vi "ELRecv.vi"(0 "connection ID":refnum<k16>) -> (2 "IP address":string, 3 "ELdata":T1, 4 "Error Out":errorcluster caption="エラー出力")   [LabVIEW 2017]
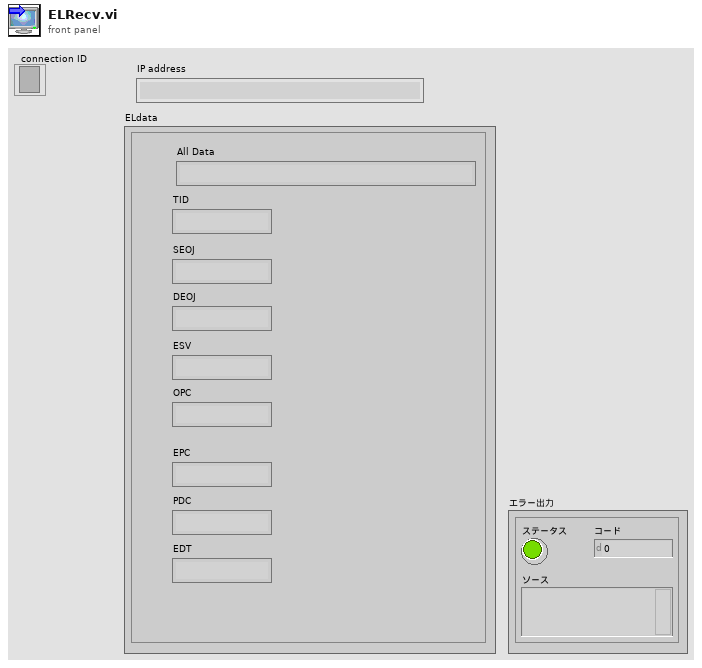
[diagram p1: front panel]
types:
  T1 = cluster{"All Data":string, "EPC":string, "EDT":string, "SEOJ":string, "DEOJ":string, "ESV":string, "OPC":string, "PDC":string, "TID":string}
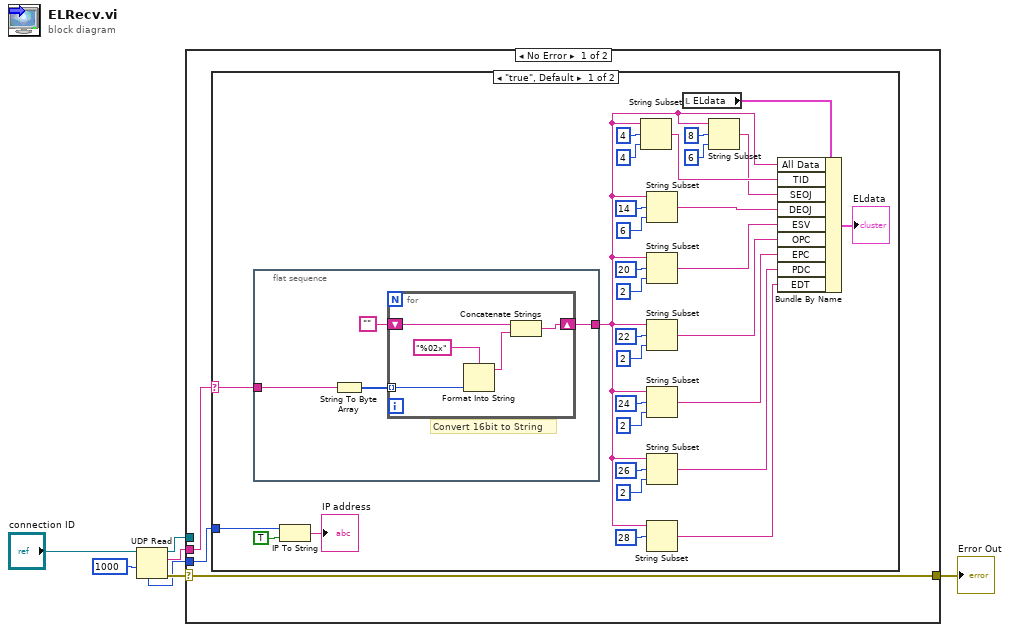
[diagram p0: block diagram]
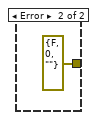
[diagram p3: hidden frame]
diagram:
  n1 = UDP Read(connection ID="connection ID", timeout ms (25000)=1000) -> (data out=w5:string, error out=w4:errorcluster, 3:w1:refnum<k16>, 6:w2:u32)  [unwired: 2 in, 1 out]
  n2 = case shown="No Error" w4 {
    selector: w4 -> [w8 _]
    tunnel: [w8 errorcluster {"status"=FALSE, "code"=0, "source"=""} ("error IO")] -> w3
    tunnel: w5 -> [w10 _]
    tunnel: w2 -> [w9 _]
    tunnel: w1 -> [_ _]
    frame No Error {
      n3 = case "ケースストラクチャ" shown="\"true\", Default" w10 {
        selector: w10 -> [w12 _]
        tunnel: w9 -> [w13 _]
        frame "true", Default {
          n4 = flat-sequence {
            tunnel: w12 -> [w42]
            tunnel: [w41] -> w11
            frame #0 {
              # "Convert 16bit to String"
              n5 = String To Byte Array(string=w42) -> (unsigned byte array=w43:u8[])
              n6 = for {
                tunnel: w43 -> [w48] mode=indexing
                shift-right: [w47] -> w41
                shift-left: "" -> [w45]
                n7 = Format Into String(format string="%02x" ("形式文字列"), w48) -> (resulting string=w46:string)  [unwired: 2 in, 1 out]
                n8 = Concatenate Strings(w45, w46) -> (w47:string)
              }
            }
          }
          n9 = IP To String(1:TRUE ("ドット表記法?（F）"), 2:w13) -> (0:→"IP address":string)
          n10 = String Subset(string=w11, offset (0)=4, length (rest)=4) -> (substring=w37:string)
          n11 = String Subset(string=w11, offset (0)=14, length (rest)=6) -> (substring=w33:string)
          n12 = String Subset(string=w11, offset (0)=20, length (rest)=2) -> (substring=w36:string)
          n13 = String Subset(string=w11, offset (0)=22, length (rest)=2) -> (substring=w34:string)
          n14 = String Subset(string=w11, offset (0)=24, length (rest)=2) -> (substring=w31:string)
          n15 = String Subset(string=w11, offset (0)=26, length (rest)=2) -> (substring=w35:string)
          n16 = String Subset(string=w11, offset (0)=28) -> (substring=w30:string)  [unwired: 1 in]
          n17 = local read "ELdata"() -> (w40:T1)
          n18 = String Subset(string=w11, offset (0)=8, length (rest)=6) -> (substring=w32:string)
          n19 = Bundle By Name(cluster=w40, "All Data"=w11, "TID"=w37, "SEOJ"=w32, "DEOJ"=w33, "ESV"=w36, "OPC"=w34, "EPC"=w31, "PDC"=w35, "EDT"=w30) -> (→"ELdata":T1)
        }
        frame "" {
        }
      }
    }
    frame Error {
    }
  }
  "Error Out" <- w3
